vi "PXI6120_Sai.vi"() -> ()   [LabVIEW 2017]
doc: "Use this template to build a producer/consumer design pattern with events to produce queue items. Use this design pattern instead of the User Interface Event Handler pattern for user interfaces when you want to execute code asynchronously in response to an event without slowing the user interface responsiveness."
uses:
  controls/FS_PXI6120sai.ctl
  hardware/PXI6251_AI/Command.ctl
panel:
  in  "Save?":bool
  in  "文件路径":path
  in  "Start/Stop":bool=TRUE
  in  "采样速率":dbl=1000.0 format="%#_6f"
  out "Waveform Graph":waveform(dbl)[](graph)
  in  "Diff_ch":T1
  # "PXI-6120模拟信号采集器"
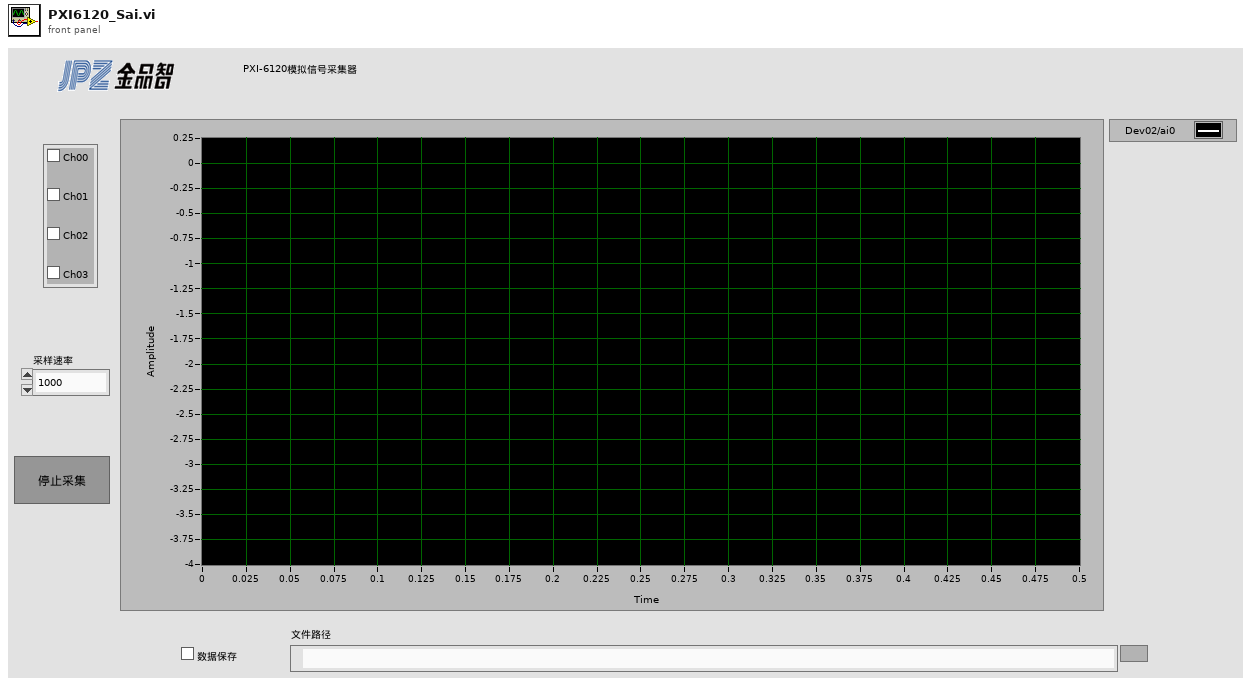
[diagram p1: front panel]
types:
  T1 = cluster{"ai00":bool, "ai01":bool, "ai02":bool, "ai03":bool}
  T2 = typedef "FS_PXI6120sai.ctl" = enum16{"Initialize", "Idel", "Start Acquire", "Read Data", "Release Daq"}
  T3 = typedef "Command.ctl" = enum16{"Start Acquire", "Read Data", "Release task"}
  T4 = cluster{"Channel":string[], "Sample rate":dbl, "input terminal configuration":i32}
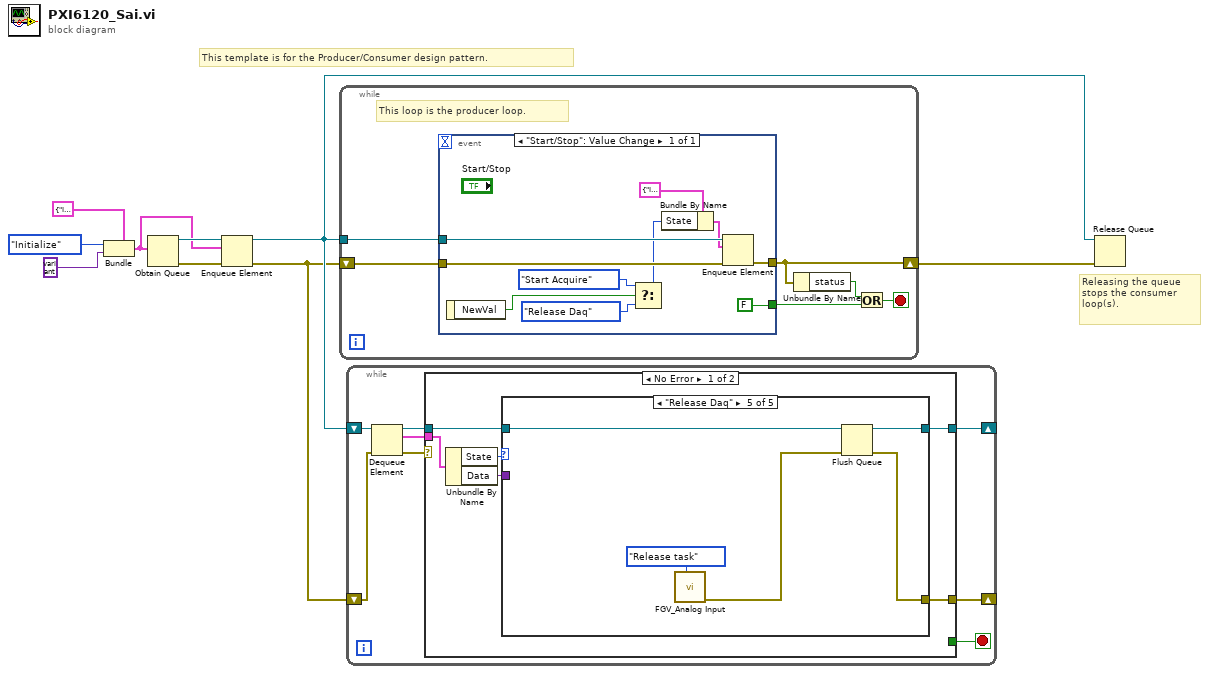
[diagram p0: block diagram]
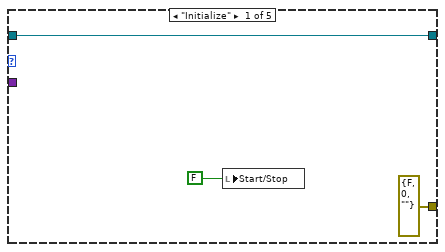
[diagram p2: hidden frame]
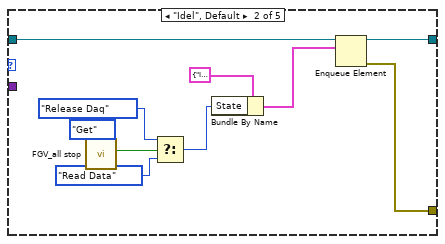
[diagram p3: hidden frame]
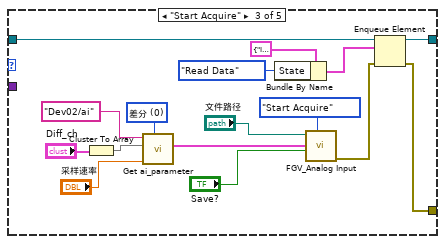
[diagram p4: hidden frame]
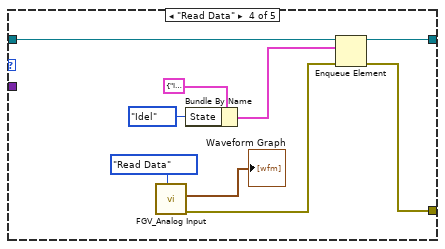
[diagram p5: hidden frame]
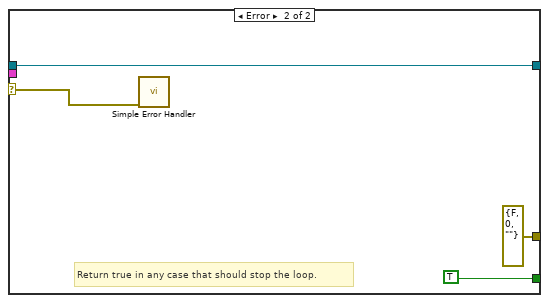
[diagram p6: hidden frame]
diagram:
  # "Releasing the queue stops the consumer loop(s)."
  # "This template is for the Producer/Consumer design pattern."
  n1 = Bundle(cluster=cluster{"State":T2, "Data":variant} {"State"=enum."Initialize", "Data"=variant}, "State"=FS_PXI6120sai."Initialize", "Data"=variant) -> (w2:cluster{"State":T2, "Data":variant})
  n2 = Obtain Queue(element data type=w2) -> (queue out=w8:refnum<queue>, error out=w4:errorcluster)  [unwired: 4 in, 1 out]
  n3 = Enqueue Element(queue=w8, element=w2, error in (no error)=w4) -> (queue out=w5:refnum<queue>, error out=w1:errorcluster)  [unwired: 1 in, 1 out]
  n4 = while {
    shift-right: [w11] -> w9
    shift-left: w1 -> [w14]
    tunnel: w5 -> [w15]
    stop <- w12 stop-if-true
    # "This loop is the producer loop."
    n5 = event shown="[0] \"Start/Stop\": Value Change" {
      selector: _ -> [_]
      dyn-events: _ -> [_]
      timeout: _ -> [_]
      tunnel: w15 -> [w25]
      tunnel: w14 -> [w24]
      tunnel: [w23] -> w11
      tunnel: [FALSE] -> w13
      event "Start/Stop": Value Change {
        n6 = event-data() -> ("NewVal"=w21:bool)  [unwired: 1 in]
        n7 = Select(t=FS_PXI6120sai."Start Acquire", s=w21, f=FS_PXI6120sai."Release Daq") -> (s? t:f=w17:T2)
        n8 = Bundle By Name(cluster=cluster{"State":T2, "Data":variant} {"State"=enum."Initialize", "Data"=variant}, "State"=w17) -> (w16:cluster{"State":T2, "Data":variant})
        n9 = Enqueue Element(queue=w25, element=w16, error in (no error)=w24) -> (error out=w23:errorcluster)  [unwired: 1 in, 2 out]
      }
    }
    n10 = Unbundle By Name(w11) -> ("status"=w10:bool)
    n11 = Or(x=w10, y=w13) -> (x .or. y?=w12:bool)
  }
  n12 = while {
    shift-right: [w27] -> _
    shift-left: w5 -> [w33]
    shift-right: [w28] -> _
    shift-left: w1 -> [w26]
    stop <- w30 stop-if-true
    n13 = Dequeue Element(queue=w33, error in (no error)=w26) -> (queue out=w29:refnum<queue>, element=w31:cluster{"State":T2, "Data":variant}, error out=w32:errorcluster)  [unwired: 1 in, 1 out]
    n14 = case shown="No Error" w32 {
      selector: w32 -> [_ w83]
      tunnel: w31 -> [w39 _]
      tunnel: [_ TRUE] -> w30
      tunnel: w29 -> [w36 w84]
      tunnel: [w35 errorcluster {"status"=FALSE, "code"=0, "source"=""} ("error out")] -> w28
      tunnel: [w34 w84] -> w27
      frame No Error {
        n15 = Unbundle By Name(w39) -> ("State"=w38:T2, "Data"=w37:variant)
        n16 = case shown="\"Release Daq\"" w38 {
          tunnel: w37 -> [_ _ _ _ _]
          tunnel: w36 -> [w41 w52 w59 w76 w81]
          tunnel: [errorcluster {"status"=FALSE, "code"=0, "source"=""} ("error out") w43 w57 w73 w78] -> w35
          tunnel: [w41 w51 w56 w75 w80] -> w34
          frame "Initialize" {
            n17 = local write "Start/Stop"(FALSE) -> ()
          }
          frame "Idel", Default {
            n18 = call "FGV_all stop.vi"("Enum"=enum16{"Set", "Get"}."Get") -> ("All Stop?"=w47:bool)  [unwired: 10 in]
            n19 = Select(t=FS_PXI6120sai."Release Daq" ("State"), s=w47, f=FS_PXI6120sai."Read Data" ("State")) -> (s? t:f=w44:T2)
            n20 = Bundle By Name(cluster=cluster{"State":T2, "Data":variant} {"State"=enum."Initialize", "Data"=variant}, "State"=w44) -> (w49:cluster{"State":T2, "Data":variant})
            n21 = Enqueue Element(queue=w52, element=w49) -> (queue out=w51:refnum<queue>, error out=w43:errorcluster)  [unwired: 2 in, 1 out]
          }
          frame "Start Acquire" {
            w68 = 0 items=["差分", "单端"] ("模式")
            n22 = Cluster To Array(cluster="Diff_ch") -> (array=w66:bool[])
            n23 = call "Get ai_parameter.vi"("模式"=w68, "采样速率"="采样速率", "Diff_ch"=w66, "Device name"="Dev02/ai") -> ("Daq_ai_para"=w61:T4)  [unwired: 7 in]
            n24 = Bundle By Name(cluster=cluster{"State":T2, "Data":variant} {"State"=enum."Initialize", "Data"=variant}, "State"=FS_PXI6120sai."Read Data") -> (w54:cluster{"State":T2, "Data":variant})
            n25 = call "FGV_Analog Input.vi"("Command"=Command."Start Acquire", "Save data?"="Save?", "Daq_ai_para"=w61, "TDMS File Path"="文件路径") -> ("error out"=w58:errorcluster)  [unwired: 5 in, 2 out]
            n26 = Enqueue Element(queue=w59, element=w54, error in (no error)=w58) -> (queue out=w56:refnum<queue>, error out=w57:errorcluster)  [unwired: 1 in, 1 out]
          }
          frame "Read Data" {
            n27 = call "FGV_Analog Input.vi"("Command"=Command."Read Data") -> ("error out"=w74:errorcluster, "data"=→"Waveform Graph":waveform(dbl)[])  [unwired: 8 in, 1 out]
            n28 = Bundle By Name(cluster=cluster{"State":T2, "Data":variant} {"State"=enum."Initialize", "Data"=variant}, "State"=FS_PXI6120sai."Idel") -> (w71:cluster{"State":T2, "Data":variant})
            n29 = Enqueue Element(queue=w76, element=w71, error in (no error)=w74) -> (queue out=w75:refnum<queue>, error out=w73:errorcluster)  [unwired: 1 in, 1 out]
          }
          frame "Release Daq" {
            n30 = call "FGV_Analog Input.vi"("Command"=Command."Release task") -> ("error out"=w79:errorcluster)  [unwired: 8 in, 2 out]
            n31 = Flush Queue(queue=w81, error in (no error)=w79) -> (queue out=w80:refnum<queue>, error out=w78:errorcluster)  [unwired: 1 out]
          }
        }
      }
      frame Error {
        # "Return true in any case that should stop the loop."
        n32 = call <vilib>:"Simple Error Handler.vi"("error in (no error)"=w83) -> ()  [unwired: 4 in, 5 out]
      }
    }
  }
  n33 = Release Queue(queue=w5, error in (no error)=w9) -> ()  [unwired: 1 in, 3 out]
